vi "GPIB_read.vi"(8 "error out 2":errorcluster, 10 "bytes":i32, 11 "GPIB Address":string) -> (0 "error out":errorcluster, 2 "data":string)   [LabVIEW 2013]
panel:
  in  "stop":bool
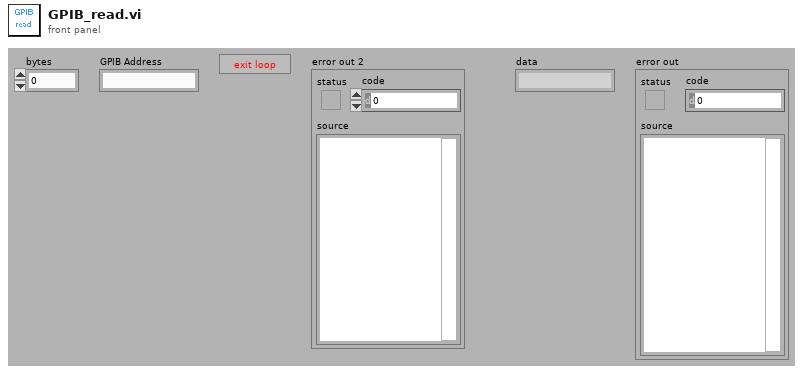
[diagram p1: front panel]
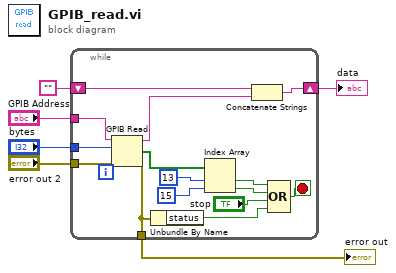
[diagram p0: block diagram]
diagram:
  n1 = while {
    tunnel: "error out 2" -> [w21]
    tunnel: "GPIB Address" -> [w20]
    tunnel: [w9] -> w5
    shift-right: [w12] -> w4
    shift-left: "" -> [w11]
    tunnel: "bytes" -> [w7]
    stop <- w18 stop-if-true
    n2 = GPIB Read(0:w20, 1:w7, 3:w21) -> (5:w10:string, 6:w17:bool[], 7:w9:errorcluster)  [unwired: 2 out]
    n3 = Unbundle By Name(w9) -> ("status"=w8:bool)
    n4 = Index Array(array=w17, index #1=13 ("index"), index #2=15 ("index")) -> (element #1=w13:bool, element #2=w14:bool)
    n5 = Concatenate Strings(w11, w10) -> (w12:string)
    n6 = Compound Arithmetic op=OR(w13, w14, "stop", w8) -> (w18:bool)
  }
  "error out" <- w5
  "data" <- w4
